vi "HGF_SVMonitor_register.vi"(0 "HGF_SVMonitor":refnum<class "HGF_SVMonitor.lvclass">, 5 "Variable URL":string, 7 "HGF_NetworkVisitor":refnum<class "HGF_NetworkVisitor.lvclass">, 9 "HGF_TriggeredEvent":refnum<class "HGF_TriggeredEvent.lvclass">, 11 "error in (no error)":errorcluster) -> (4 "HGF_SVMonitor":refnum<class "HGF_SVMonitor.lvclass">, 15 "error out":errorcluster)   [LabVIEW 2012, in "HGF_SV.lvlib" / "HGF_SVMonitor.lvclass"]
doc: "Executes command \"register\""
uses:
  HGF_SVMonitor.lvclass
  HGF_BaseClasses/HGF_NetworkVisitor/HGF_NetworkVisitor.lvclass
  HGF_BaseClasses/HGF_TriggeredEvent/HGF_TriggeredEvent.lvclass
  HGF_SVMonitor.lvclass/HGF_SVMonitor.ctl
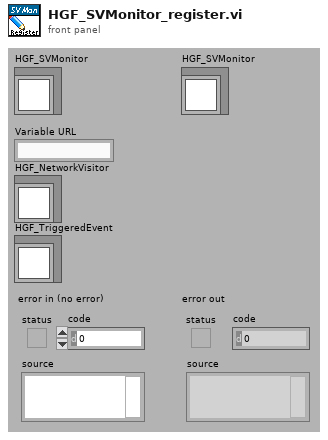
[diagram p1: front panel]
types:
  T1 = cluster{"registered Visitors":cluster{"HGF_NetworkVisitor":refnum<class "HGF_NetworkVisitor.lvclass">, "HGF_TriggeredEvent":refnum<class "HGF_TriggeredEvent.lvclass">}[], "last known data":variant, "Time Stamp":timestamp, "shared variable refnum in":refnum<k21>}
  T2 = cluster{"registered Visitors":cluster{"HGF_NetworkVisitor":refnum<class "HGF_NetworkVisitor.lvclass">, "HGF_TriggeredEvent":refnum<class "HGF_TriggeredEvent.lvclass">}[], "last known data":variant, "Time Stamp":timestamp, "shared variable refnum in":refnum<k21>}[]
  T3 = cluster{"HGF_NetworkVisitor":refnum<class "HGF_NetworkVisitor.lvclass">, "HGF_TriggeredEvent":refnum<class "HGF_TriggeredEvent.lvclass">}
  T4 = cluster{"HGF_NetworkVisitor":refnum<class "HGF_NetworkVisitor.lvclass">, "HGF_TriggeredEvent":refnum<class "HGF_TriggeredEvent.lvclass">}[]
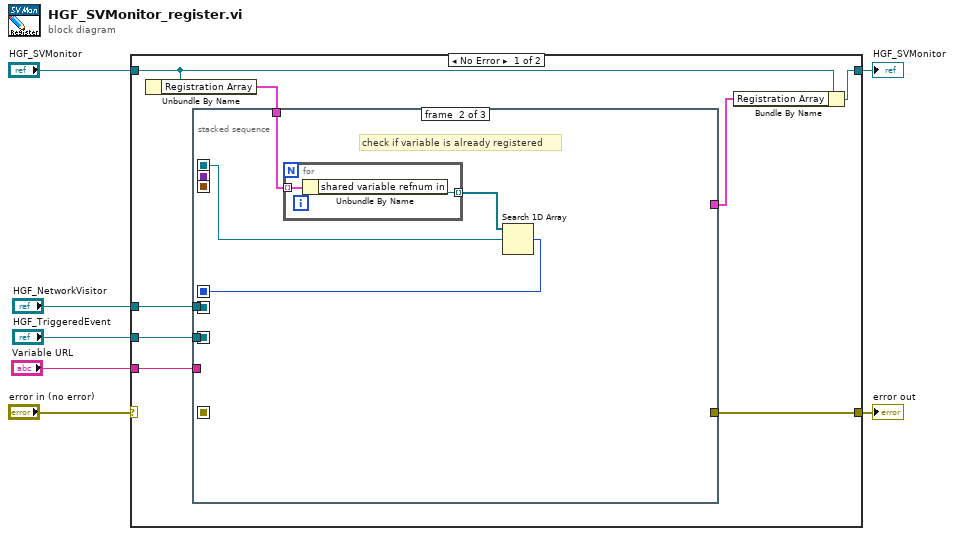
[diagram p0: block diagram]
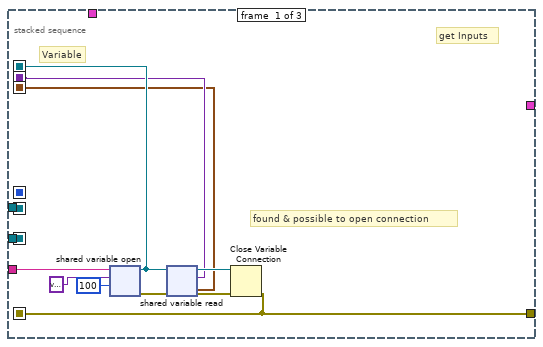
[diagram p2: hidden frame]
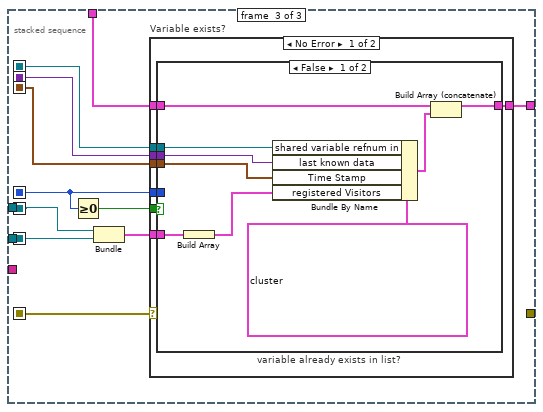
[diagram p3: hidden frame]
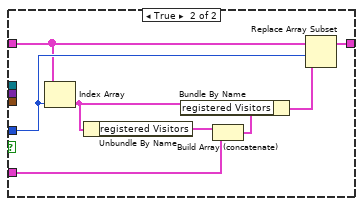
[diagram p4: hidden frame]
diagram:
  n1 = case shown="No Error" "error in (no error)" {
    selector: "error in (no error)" -> [_ w71]
    tunnel: [w9 w71] -> w6
    tunnel: [w13 w72] -> w4
    tunnel: "HGF_SVMonitor" -> [w14 w72]
    tunnel: "Variable URL" -> [w11 _]
    tunnel: "HGF_NetworkVisitor" -> [w8 _]
    tunnel: "HGF_TriggeredEvent" -> [w10 _]
    frame No Error {
      n2 = Unbundle By Name(w14) -> ("Registration Array"=w15:T2)
      n3 = stacked-sequence {
        seq-local: [_ w28 _] -> [_ _ w43]
        seq-local: [w18 _ _] -> [_ _ w37]
        seq-local: [w25 _ _] -> [_ w29 w40]
        seq-local: [w17 _ _] -> [_ _ w39]
        seq-local: [w21 _ _] -> [_ _ w36]
        seq-local: [w20 _ _] -> [_ _ w35]
        seq-local: [w16 _ _] -> [_ _ w34]
        tunnel: w15 -> [_ w31 w42]
        tunnel: [_ _ w41] -> w12
        tunnel: w11 -> [w27 _ _]
        tunnel: w10 -> [w17 _ _]
        tunnel: [w18 _ _] -> w9
        tunnel: w8 -> [w16 _ _]
        frame #0 {
          # "Variable"
          # "found & possible to open connection"
          # "get Inputs"
          n4 = shared-variable-open(w27, variant ("variant"), 100 ("timeout ms")) -> (w25:refnum<k21>, w23:errorcluster)  [unwired: 3 in]
          n5 = shared-variable-read(w25, w23) -> (w24:refnum<k21>, w22:errorcluster, w21:variant, w20:timestamp)
          n6 = Close Variable Connection(8:w22, 11:w24) -> (0:w18:errorcluster)
        }
        frame #1 {
          # "check if variable is already registered"
          n7 = for {
            tunnel: w31 -> [w33] mode=indexing
            tunnel: [w32] -> w30 mode=indexing
            n8 = Unbundle By Name(w33) -> ("shared variable refnum in"=w32:refnum<k21>)
          }
          n9 = Search 1D Array(1D array=w30, element=w29) -> (index of element=w28:i32)  [unwired: 1 out]
        }
        frame #2 {
          n10 = Greater Or Equal To 0?(x=w43) -> (x >= 0?=w44:bool)
          n11 = Bundle("HGF_NetworkVisitor"=w34, "HGF_TriggeredEvent"=w39) -> (w38:T3)  [unwired: 1 out]
          n12 = case "Variable exists?" shown="No Error" w37 {
            tunnel: w44 -> [w52 _]
            tunnel: w43 -> [w51 _]
            tunnel: w42 -> [w50 w70]
            tunnel: [w49 w70] -> w41
            tunnel: w40 -> [w48 _]
            tunnel: w38 -> [w47 _]
            tunnel: w36 -> [w46 _]
            tunnel: w35 -> [w45 _]
            frame No Error {
              n13 = case "variable already exists in list?" shown="False" w52 {
                tunnel: w51 -> [_ w66]
                tunnel: w50 -> [w58 w65]
                tunnel: [w61 w63] -> w49
                tunnel: w48 -> [w59 _]
                tunnel: w47 -> [w60 w62]
                tunnel: w46 -> [w56 _]
                tunnel: w45 -> [w55 _]
                frame False {
                  n14 = Build Array(w60) -> (w54:T4)
                  n15 = Bundle By Name(cluster=T1 {"registered Visitors"=[], "last known data"=variant, "Time Stamp"=timestamp(0 s since 1904-01-01), "shared variable refnum in"=""} ("element"), "shared variable refnum in"=w59, "last known data"=w56, "Time Stamp"=w55, "registered Visitors"=w54) -> (w53:T1)
                  n16 = Build Array (concatenate)(w58, w53) -> (w61:T2)
                }
                frame True {
                  n17 = Index Array(array=w65, index=w66) -> (element=w68:T1)
                  n18 = Unbundle By Name(w68) -> ("registered Visitors"=w69:T4)
                  n19 = Build Array (concatenate)(w69, w62) -> (w67:T4)
                  n20 = Bundle By Name(cluster=w68, "registered Visitors"=w67) -> (w64:T1)
                  n21 = Replace Array Subset(array=w65, new element=w64, index=w66) -> (w63:T2)
                }
              }
            }
            frame Error {
            }
          }
        }
      }
      n22 = Bundle By Name(cluster=w14, "Registration Array"=w12) -> (w13:refnum<class "HGF_SVMonitor.lvclass">)
    }
    frame Error {
    }
  }
  "error out" <- w6
  "HGF_SVMonitor" <- w4
